vi "Resolve Symbolic Path.vi"(9 "Component Root Path":path, 10 "Path In":path) -> (1 "error out":errorcluster, 2 "Path Out":path)   [LabVIEW 2017, in "CL_G3_VIComponentBuilder.lvlib"]
doc: "Resolves any symbolic path in the given path input by expanding it to a full pathname.\n\nSymbolic Paths supported:\n<ComponetBuilderSourceDir>—Referes to the source directory of the component builder.\n<ComponentDef>—Refers to the directory containing the component's \"Component Definition.ini\" File\n<vilib>—Refers to the vi.lib directory in the labview directory. \n<userlib>—Refers to the user.lib directory in the labview directory. \n<instrlib>—Refers to the instr.lib directory in the labview directory. \n<helpdir>—Refers to the help directory in the labview directory."
uses:
  CL_G3_VIComponentBuilder.lvlib
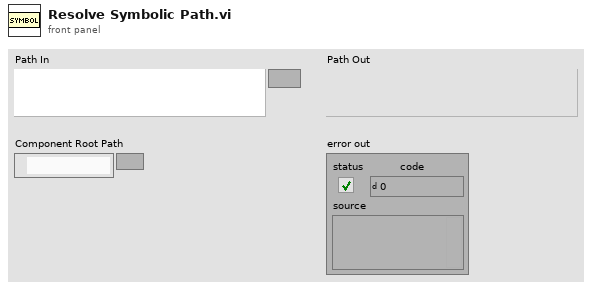
[diagram p1: front panel]
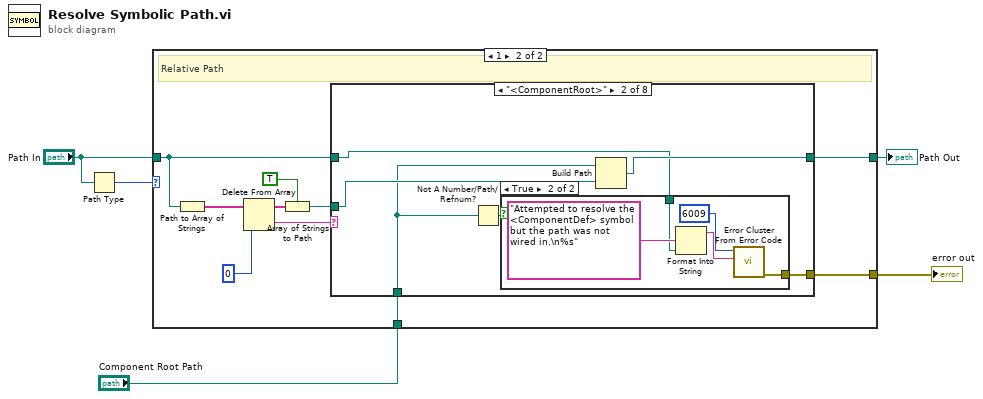
[diagram p0: block diagram]
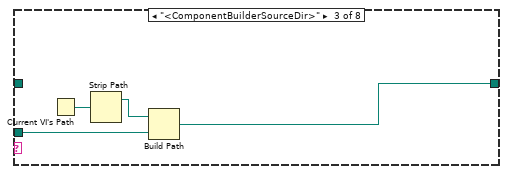
[diagram p5: hidden frame]
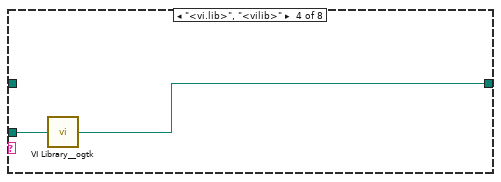
[diagram p6: hidden frame]
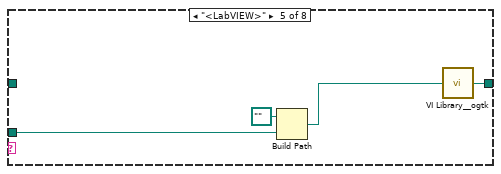
[diagram p7: hidden frame]
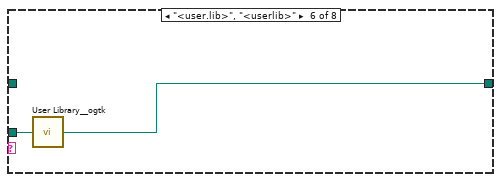
[diagram p8: hidden frame]
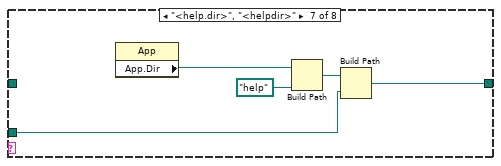
[diagram p9: hidden frame]
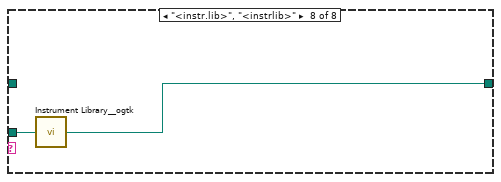
[diagram p10: hidden frame]
diagram:
  n1 = Path Type(1:"Path In") -> (0:w5:i16)
  n2 = case shown="1" w5 {
    tunnel: "Path In" -> [w6 w10]
    tunnel: [w6 w11] -> w3
    tunnel: [_ w8] -> w2
    tunnel: "Component Root Path" -> [_ w7]
    frame 0, Default {
      # "0-Absolute Path; 2-Not a path"
    }
    frame 1 {
      # "Relative Path"
      n3 = Path to Array of Strings(0:w10) -> (2:w16:string[])  [unwired: 1 out]
      n4 = Delete From Array(array=w16, index=0) -> (deleted portion=w15:string, array with subset deleted=w13:string[])  [unwired: 1 in]
      n5 = Array of Strings to Path(0:w13, 1:TRUE ("relative")) -> (2:w12:path)
      n6 = case shown="\"<ComponentRoot>\"" w15 {
        tunnel: w12 -> [_ w22 w31 w34 w35 w40 w43 w47]
        tunnel: [w17 w23 w29 w33 w38 w39 w41 w46] -> w11
        tunnel: w10 -> [w17 w20 _ _ _ _ _ _]
        tunnel: [_ w19 _ _ _ _ _ _] -> w8
        tunnel: w7 -> [_ w18 _ _ _ _ _ _]
        frame "False", Default {
        }
        frame "<ComponentRoot>" {
          n7 = Not A Number/Path/Refnum?(number/path/refnum=w18) -> (NaN/Path/Refnum?=w21:bool)
          n8 = case shown="True" w21 {
            tunnel: w20 -> [_ w27]
            tunnel: [_ w24] -> w19
            frame False {
            }
            frame True {
              n9 = Format Into String(format string="Attempted to resolve the <ComponentDef> symbol but the path was not wired in.\n%s", w27) -> (resulting string=w26:string)  [unwired: 2 in, 1 out]
              n10 = call <vilib>:"Error Cluster From Error Code.vi"("error message (\"\")"=w26, "error code (0)"=6009) -> ("error out"=w24:errorcluster)  [unwired: 7 in]
            }
          }
          n11 = Build Path(base path=w18, name or relative path=w22) -> (appended path=w23:path)
        }
        frame "<ComponentBuilderSourceDir>" {
          n12 = Current VI's Path() -> (path=w32:path)
          n13 = Strip Path(path=w32) -> (stripped path=w30:path)  [unwired: 1 out]
          n14 = Build Path(base path=w30, name or relative path=w31) -> (appended path=w29:path)
        }
        frame "<vi.lib>", "<vilib>" {
          n15 = call <userlib>:"VI Library__ogtk.vi"("Relative path (.)"=w34) -> ("VI Library (+ Relative)"=w33:path)
        }
        frame "<LabVIEW>" {
          n16 = Build Path(base path=path ".." ("Relative path (.)"), name or relative path=w35) -> (appended path=w36:path)
          n17 = call <userlib>:"VI Library__ogtk.vi"("Relative path (.)"=w36) -> ("VI Library (+ Relative)"=w38:path)
        }
        frame "<user.lib>", "<userlib>" {
          n18 = call <userlib>:"User Library__ogtk.vi"("Relative path (.)"=w40) -> ("User Library (+ Relative)"=w39:path)
        }
        frame "<help.dir>", "<helpdir>" {
          n19 = property class="App"() -> ("App.Dir"=w45:path)  [unwired: 2 in, 2 out]
          n20 = Build Path(base path=w45, name or relative path=path "help") -> (appended path=w42:path)
          n21 = Build Path(base path=w42, name or relative path=w43) -> (appended path=w41:path)
        }
        frame "<instr.lib>", "<instrlib>" {
          n22 = call <userlib>:"Instrument Library__ogtk.vi"("Relative path (.)"=w47) -> ("Instrument Library (+ Relative)"=w46:path)
        }
      }
    }
  }
  "Path Out" <- w3
  "error out" <- w2
